vi "EverybotHang Handler.vi"(11 "JoystickDevRef":T1={"Device"=enum."USB 1"}) -> ()   [LabVIEW 2019]
uses:
  <vilib>/Rock Robotics/WPI/Joystick/WPI_JoystickDevRef.ctl
  <vilib>/Rock Robotics/WPI/Joystick/WPI_JoystickDeviceEnum.ctl
  EverybotHang Operations.ctl
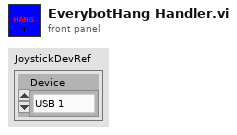
[diagram p1: front panel]
types:
  T1 = typedef "WPI_JoystickDevRef.ctl" = cluster{"Device":T2}
  T2 = typedef "WPI_JoystickDeviceEnum.ctl" = enum16{"USB 0", "USB 1", "USB 2", "USB 3", "USB 4", "USB 5"}
  T3 = typedef "EverybotHang Operations.ctl" = enum16{"Reserve", "Read Current", "Immediate", "Immediate Reverse"}
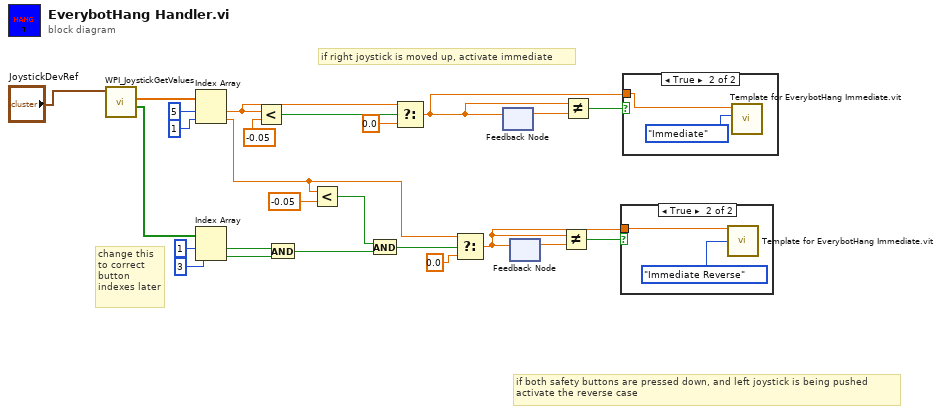
[diagram p0: block diagram]
diagram:
  # "if both safety buttons are pressed down, and left joystick is being pushed\nactivate the reverse case"
  # "if right joystick is moved up, activate immediate"
  # "change this\nto correct\nbutton\nindexes later"
  n1 = call <vilib>:"WPI_JoystickGetValues.vi"("JoystickDevRef"="JoystickDevRef") -> ("Buttons"=w17:bool[], "Axes"=w22:dbl[])  [unwired: 6 in, 3 out]
  n2 = Index Array(array=w22, index #1=5 ("index"), index #2=1 ("index")) -> (element #1=w20:dbl, element #2=w7:dbl)
  n3 = Index Array(array=w17, index #1=1 ("index"), index #2=3 ("index")) -> (element #1=w14:bool, element #2=w13:bool)
  n4 = Less?(x=w20, y=-0.05) -> (x < y?=w21:bool)
  n5 = And(x=w14, y=w13) -> (x .and. y?=w9:bool)
  n6 = Less?(x=w7, y=-0.05) -> (x < y?=w10:bool)
  n7 = And(x=w10, y=w9) -> (x .and. y?=w8:bool)
  n8 = Select(t=w20, s=w21, f=0.0) -> (s? t:f=w1:dbl)
  n9 = Select(t=w7, s=w8, f=0.0) -> (s? t:f=w4:dbl)
  n10 = feedback-in #1(w1) -> ()
  n11 = feedback #1() -> (w3:dbl)  [unwired: 1 in]
  n12 = feedback-in #2(w4) -> ()
  n13 = feedback #2() -> (w6:dbl)  [unwired: 1 in]
  n14 = Not Equal?(x=w4, y=w6) -> (x != y?=w5:bool)
  n15 = Not Equal?(x=w1, y=w3) -> (x != y?=w2:bool)
  n16 = case shown="True" w5 {
    tunnel: w4 -> [_ w26]
    frame False {
    }
    frame True {
      n17 = call "Template for EverybotHang Immediate.vit"("Operation"=EverybotHang_Operations."Immediate Reverse", "Setpoint"=w26) -> ()  [unwired: 9 in, 1 out]
    }
  }
  n18 = case shown="True" w2 {
    tunnel: w1 -> [_ w28]
    frame False {
    }
    frame True {
      n19 = call "Template for EverybotHang Immediate.vit"("Operation"=EverybotHang_Operations."Immediate", "Setpoint"=w28) -> ()  [unwired: 9 in, 1 out]
    }
  }
